vi "Read Generic Data Frame from TCP.vi"(8 "error in (no error)":errorcluster, 11 "TCP Network Connection in":refnum<k5>) -> (0 "error out":errorcluster, 1 "Valid CRC":bool, 2 "Frame Received":T1 {"CRC" format="%08x"; "Frame Header"."Options" format="%016b"; "Frame Header"."Time" format="%^<%I:%M:%S%3u %p\n%m/%d/%Y %Z>T"; "Frame Header"."Sync" format="%08x"}, 3 "TCP Network Connection out":refnum<k5>)   [LabVIEW 2023]
uses:
  Type Definitions/Data Frame.ctl
  Type Definitions/Data Frame Header.ctl
  Type Definitions/Payload Class.ctl
  Type Definitions/Device.ctl
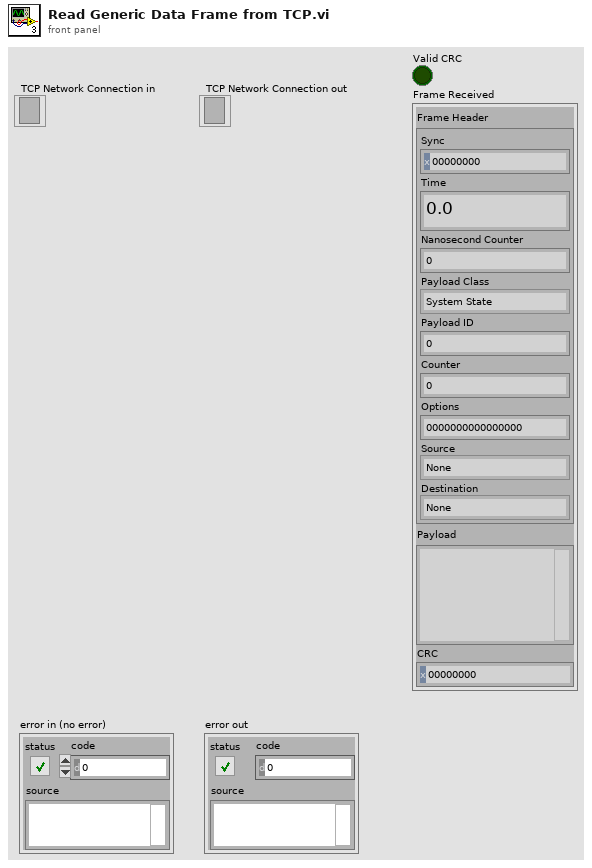
[diagram p1: front panel]
types:
  T1 = typedef "Data Frame.ctl" = cluster{"Frame Header":T2, "Payload":string, "CRC":u32}
  T2 = typedef "Data Frame Header.ctl" = cluster{"Sync":u32, "Time":dbl, "Nanosecond Counter":i64, "Payload Class":T3, "Payload ID":u16, "Counter":i32, "Options":u32, "Source":T4, "Destination":T4}
  T3 = typedef "Payload Class.ctl" = enum16{"System State", "Parameters", "Metadata", "Software Monitor", "Data", "Commands"}
  T4 = typedef "Device.ctl" = enum32{"None", "Exec", "Aux1", "Aux2", "Aux3"}
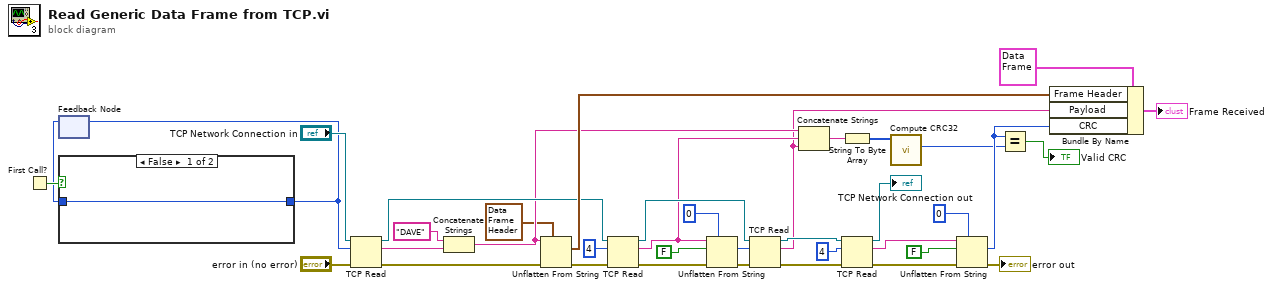
[diagram p0: block diagram]
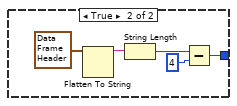
[diagram p2: hidden frame]
diagram:
  n1 = First Call?() -> (First Call?: T/F=w3:bool)
  n2 = feedback #1() -> (w2:i32)  [unwired: 1 in]
  n3 = case shown="False" w3 {
    tunnel: [w39 w40] -> w1
    tunnel: w2 -> [w39 _]
    frame False {
    }
    frame True {
      n4 = Flatten To String(anything=T2 {"Sync"=0, "Time"=0.0, "Nanosecond Counter"=0, "Payload Class"=enum."System State", "Payload ID"=0, "Counter"=0, "Options"=0, "Source"=enum."None", "Destination"=enum."None"} ("Frame Header")) -> (data string=w43:string)  [unwired: 3 in, 2 out]
      n5 = String Length(string=w43) -> (length=w44:i32)
      n6 = Subtract(x=w44, y=4) -> (x-y=w40:i32)
    }
  }
  n7 = feedback-in #1(w1) -> ()
  n8 = TCP Read(connection ID="TCP Network Connection in", bytes to read=w1, error in (no error)="error in (no error)") -> (connection ID out=w16:refnum<k5>, data out=w30:string, error out=w35:errorcluster)  [unwired: 2 in]
  n9 = Concatenate Strings("DAVE" ("string"), w30) -> (w14:string)
  n10 = Unflatten From String(type=T2 {"Sync"=0, "Time"=0.0, "Nanosecond Counter"=0, "Payload Class"=enum."System State", "Payload ID"=0, "Counter"=0, "Options"=0, "Source"=enum."None", "Destination"=enum."None"} ("Frame Header"), binary string=w14, error in (no error)=w35) -> (value=w22:T2, error out=w36:errorcluster)  [unwired: 2 in, 1 out]
  n11 = TCP Read(connection ID=w16, bytes to read=4, error in (no error)=w36) -> (connection ID out=w21:refnum<k5>, data out=w13:string, error out=w32:errorcluster)  [unwired: 2 in]
  n12 = Unflatten From String(type=0 ("bytes to read"), binary string=w13, data includes array or string size? (T)=FALSE, error in (no error)=w32) -> (value=w20:i32, error out=w33:errorcluster)  [unwired: 1 in, 1 out]
  n13 = TCP Read(connection ID=w21, bytes to read=w20, error in (no error)=w33) -> (connection ID out=w23:refnum<k5>, data out=w12:string, error out=w34:errorcluster)  [unwired: 2 in]
  n14 = Concatenate Strings(w14, w13, w12) -> (w11:string)
  n15 = String To Byte Array(string=w11) -> (unsigned byte array=w10:u8[])
  n16 = TCP Read(connection ID=w23, bytes to read=4, error in (no error)=w34) -> (connection ID out=→"TCP Network Connection out":refnum<k5>, data out=w27:string, error out=w37:errorcluster)  [unwired: 2 in]
  n17 = call "Compute CRC32.vi"("inputArray"=w10) -> ("CRC32Value"=w8:u32)  [unwired: 9 in, 1 out]
  n18 = Unflatten From String(type=u32 0 ("bytes to read"), binary string=w27, data includes array or string size? (T)=FALSE, error in (no error)=w37) -> (value=w9:u32, error out=→"error out":errorcluster)  [unwired: 1 in, 1 out]
  n19 = Equal?(x=w9, y=w8) -> (x = y?=→"Valid CRC":bool)
  n20 = Bundle By Name(cluster=T1 {"Frame Header"={"Sync"=0, "Time"=0.0, "Nanosecond Counter"=0, "Payload Class"=enum."System State", "Payload ID"=0, "Counter"=0, "Options"=0, "Source"=enum."None", "Destination"=enum."None"}, "Payload"="", "CRC"=0} ("Frame"), "Frame Header"=w22, "Payload"=w12, "CRC"=w9) -> (→"Frame Received":T1)
